vi "RF Test.vi"(0 "instrument handle":refnum<k15>, 2 "No Reverse":bool, 3 "file name":string, 5 "Num of Frames":i32, 9 "Num of Vectors":i32, 11 "error out":errorcluster) -> ()   [LabVIEW 2022 SP3]
uses:
  Motion Controllers/-MotionRoutines/MotionGlobals.vi
  <vilib>/Platform/TimedLoop/XDataNode/XDataNode.xnode
  <vilib>/Platform/TimedLoop/XDataNode/nitl_modes.ctl
  <vilib>/Platform/TimedLoop/XDataNode/XDNodeRunTimeDep.lvlib
  <vilib>/Platform/TimedLoop/XDataNode/wakeup.ctl
  <vilib>/Platform/TimedLoop/XDataNode/timing_clust.ctl
  <instrlib>/niScope/Acquire/Fetch/niScope Multi Fetch Binary 8.vi
  -ScanSystem/DataHandling/ReverseDataI8.vi
  Acqiris/-AcqirisRoutines/VScaleInfoAcq.vi
panel:
  in  "instrument handle 3":refnum<k15>
  out "x-y":u32
  out "result":i32
  in  "instrument handle 2":refnum<k15>
  out "frame time":u32
  out "Records Done":i32
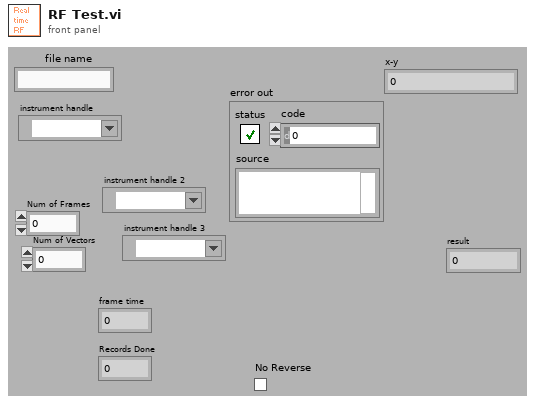
[diagram p1: front panel]
types:
  T1 = typedef "XDNodeRunTimeDep.lvlib/timing_clust.ctl" = cluster{"Expected End [f-1]":u64, "Actual End [f-1]":u64, "Finished Late? [f-1]":bool, "Expected End [i-1]":u64, "Actual End [i-1]":u64, "Finished Late? [i-1]":bool, "Expected Start [i]":u64, "Actual Start [i]":u64, "Expected Start [f]":u64, "Actual Start [f]":u64, "Source Name":string, "Structure Name":string, "Period":i64, "Deadline":i64, "Offset":i64, "Start":i64, "Priority":i32, "Timeout":i32, "Mode":T2, "Wakeup Reason":T3, "Error":errorcluster, "Source Type":string, "Secondary Source Type":string, "Global End Time":u64, "Global Start Time":u64, "Frame Duration":u64, "Iteration Duration":u64, "Assigned CPU":i32, "I/O Scan Engine Mode":u32}
  T2 = typedef "XDNodeRunTimeDep.lvlib/nitl_modes.ctl" = enum32{"No Change", "Process missed periods, maintain original phase", "Discard missed periods, maintain original phase", "Process missed periods, ignore original phase", "Discard missed periods, ignore original phase"}
  T3 = typedef "XDNodeRunTimeDep.lvlib/wakeup.ctl" = enum32{"Normal", "Aborted", "Asynchronous wakeup", "Timing source error", "Timed loop error", "Timeout"}
  T4 = cluster{sgl, "Gain [dB]  ":sgl, "Atten (dB)":sgl}
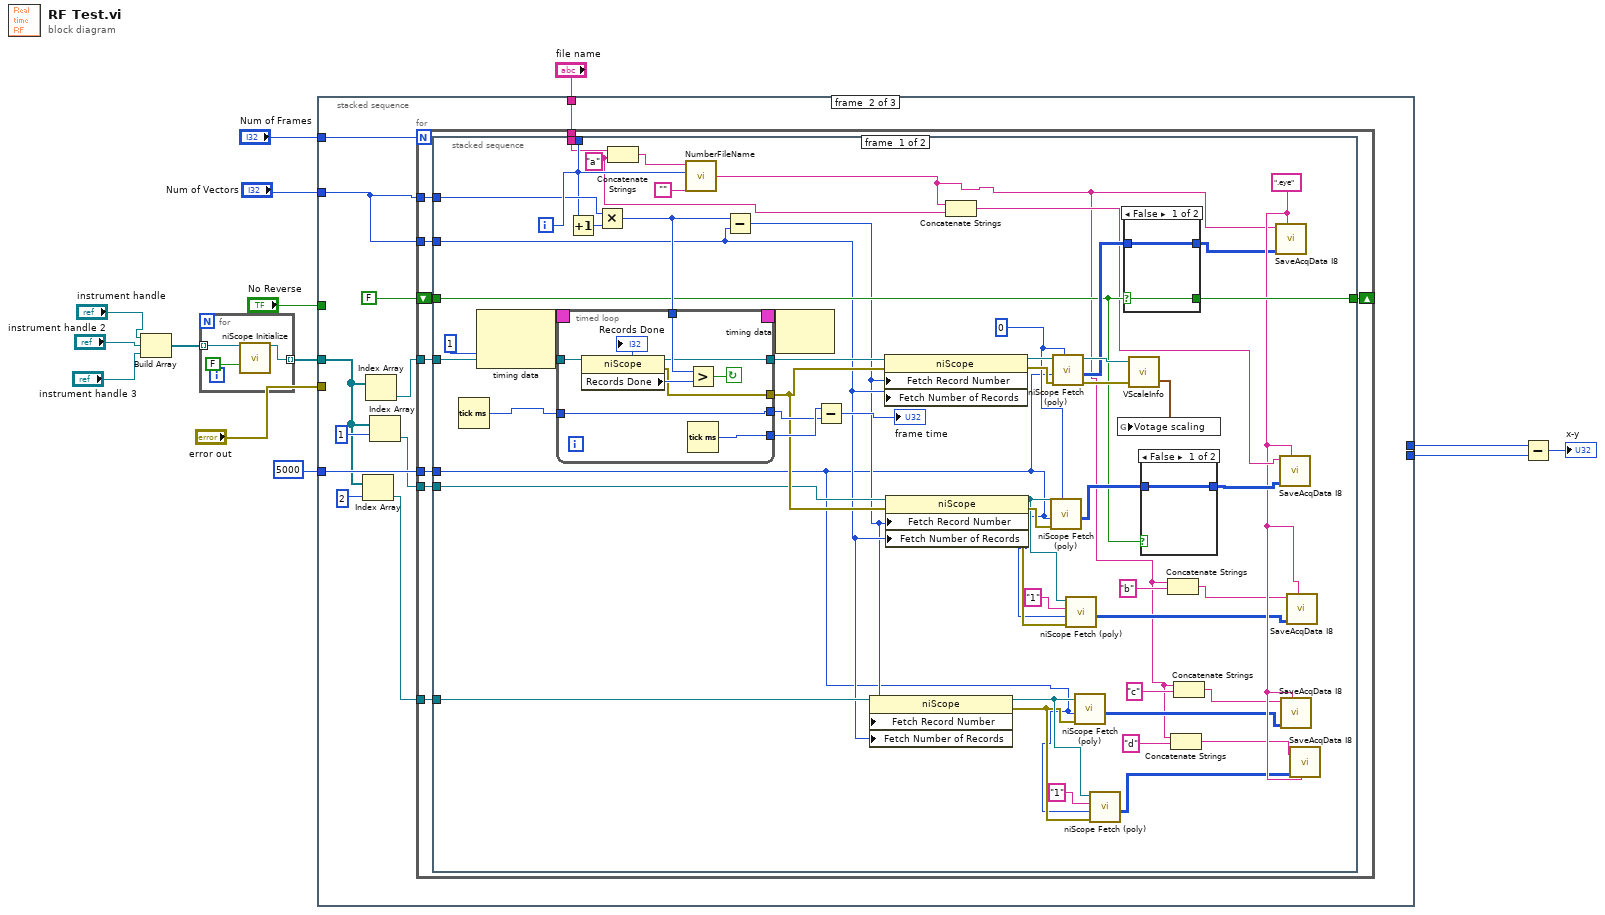
[diagram p0: block diagram]
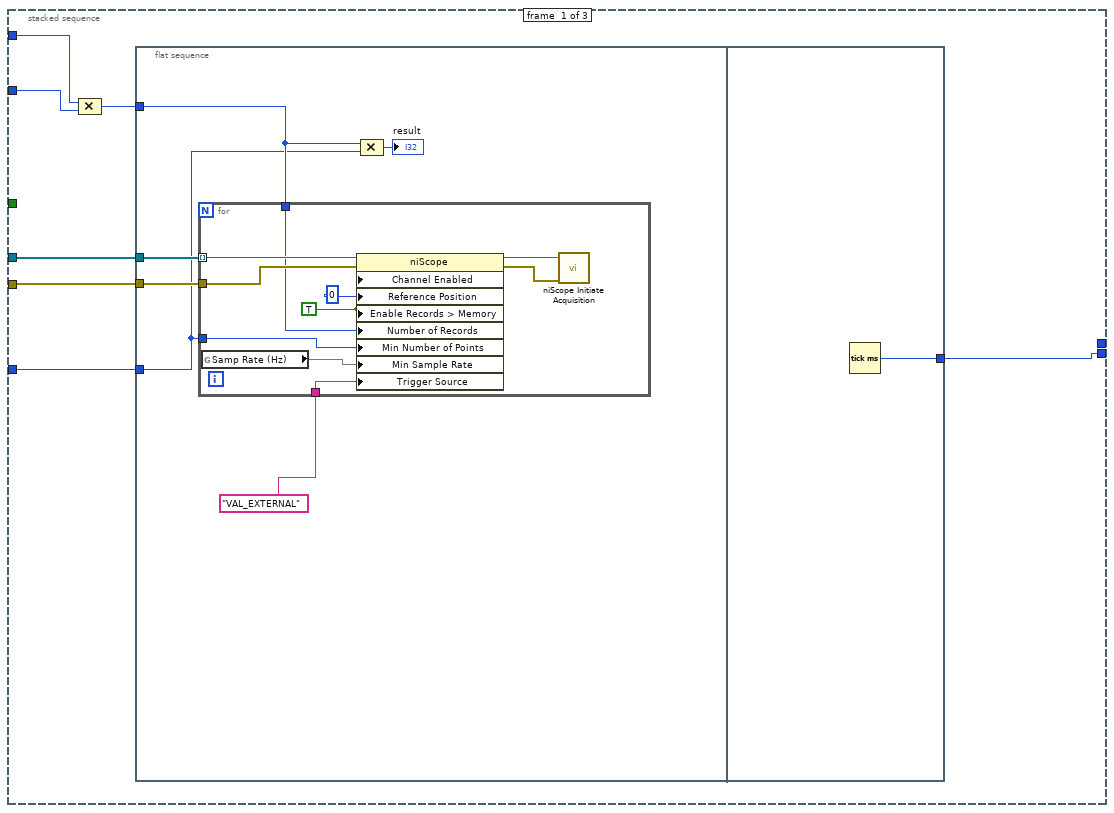
[diagram p2: hidden frame]
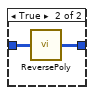
[diagram p3: hidden frame]
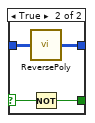
[diagram p4: hidden frame]
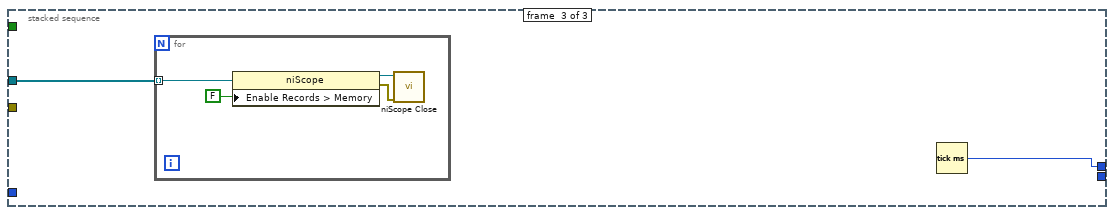
[diagram p6: hidden frame]
diagram:
  n1 = Build Array("instrument handle", "instrument handle 2", "instrument handle 3") -> (w2:refnum<k15>[])
  n2 = for {
    tunnel: [w17] -> w8 mode=indexing
    tunnel: w2 -> [w15] mode=indexing
    n3 = call <instrlib>:"niScope Initialize.vi"("resource name"=w15, "reset device"=FALSE) -> ("instrument handle"=w17:refnum<k15>)  [unwired: 2 in, 11 out]
  }
  n4 = stacked-sequence {
    tunnel: "error out" -> [w24 _ _]
    tunnel: w8 -> [w23 w44 w140]
    tunnel: "Num of Frames" -> [w22 w51 _]
    tunnel: "Num of Vectors" -> [w21 w48 _]
    tunnel: 5000 ("rf points per line") -> [w19 w52 _]
    tunnel: "file name" -> [_ w50 _]
    tunnel: "No Reverse" -> [_ _ _]
    tunnel: [_ _ w139] -> w7
    tunnel: [w18 _ _] -> w6
    frame #0 {
      n5 = Compound Arithmetic op=MULTIPLY(w22, w21) -> (w20:i32)
      n6 = flat-sequence {
        tunnel: w24 -> [w30]
        tunnel: w23 -> [w29]
        tunnel: w20 -> [w27]
        tunnel: w19 -> [w26]
        tunnel: [w41] -> w18
        frame #0 {
          n7 = for {
            tunnel: w30 -> [w39]
            tunnel: w29 -> [w38] mode=indexing
            tunnel: "VAL_EXTERNAL" ("Triggering:Trigger Source") -> [w33]
            tunnel: w27 -> [w32]
            tunnel: w26 -> [w31]
            w36 = TRUE ("Horizontal:Enable Records > Memory")
            n8 = global read "MotionGlobals.vi" "Samp Rate (Hz)"() -> (w34)
            n9 = property class="niScope"(reference=w38, error in=w39, "Channel Enabled"=w36, "Reference Position"=0, "Enable Records > Memory"=w36, "Number of Records"=w32, "Min Number of Points"=w31, "Min Sample Rate"=w34, "Trigger Source"=w33) -> (reference out=w40:refnum<k15>, error out=w37:errorcluster)
            n10 = call <instrlib>:"niScope Initiate Acquisition.vi"("instrument handle"=w40, "error in"=w37) -> ()  [unwired: 14 out]
          }
          n11 = Compound Arithmetic op=MULTIPLY(w27, w26) -> (→"result":i32)
        }
        frame #1 {
          n12 = Tick Count (ms)() -> (millisecond timer value=w41:u32)
        }
      }
    }
    frame #1 {
      n13 = Index Array(array=w44, index=2) -> (element=w42:refnum<k15>)
      n14 = Index Array(array=w44) -> (element=w47:refnum<k15>)  [unwired: 1 in]
      n15 = Index Array(array=w44, index=1) -> (element=w43:refnum<k15>)
      n16 = for {
        N: w51 -> [_]
        tunnel: w52 -> [w55]
        tunnel: w47 -> [w62]
        tunnel: w48 -> [w61]
        tunnel: w48 -> [w57]
        tunnel: w50 -> [w59]
        shift-right: [w58] -> _
        shift-left: FALSE -> [w56]
        tunnel: w43 -> [w54]
        tunnel: w42 -> [w53]
        i -> [w60]
        n17 = stacked-sequence {
          tunnel: w62 -> [w111 _]
          tunnel: w61 -> [w109 _]
          tunnel: w60 -> [w103 _]
          tunnel: w59 -> [w101 _]
          tunnel: [w98 _] -> w58
          tunnel: w57 -> [w80 _]
          tunnel: w56 -> [w92 _]
          tunnel: w55 -> [w78 _]
          tunnel: w54 -> [w84 _]
          tunnel: w53 -> [w81 _]
          frame #0 {
            w90 = 0
            w71 = ".eye" ("Ext")
            w91 = "a"
            n18 = Tick Count (ms)() -> (millisecond timer value=w88:u32)
            n19 = node-c288(i64 1 ("Period")) -> (w115:T1)  [unwired: 1 out]
            n20 = Increment(x=w103) -> (x+1=w110:i32)
            n21 = Multiply(x=w109, y=w110) -> (x*y=w106:i32)
            n22 = timed-loop {
              tunnel: w111 -> [w132]
              tunnel: w106 -> [w131]
              tunnel: [w129] -> w108
              tunnel: [w127] -> w89
              timing: w115 -> [_]
              timing-out: [_] -> w114
              tunnel: [w126] -> w95
              tunnel: w88 -> [w126]
              tunnel: [w125] -> w96
              stop <- w130 continue-if-true
              n23 = property class="niScope"(reference=w132) -> (reference out=w129:refnum<k15>, error out=w127:errorcluster, "Records Done"=w128:i32)  [unwired: 1 in]
              "Records Done" <- w128
              n24 = Greater?(x=w131, y=w128) -> (0:w130:bool)
              n25 = Tick Count (ms)() -> (millisecond timer value=w125:u32)
            }
            n26 = Concatenate Strings(w101, w91) -> (w100:string)
            n27 = call "NumberFileName.vi"("String"="", "File number"=w103, "file name"=w100) -> ("Numbered File"=w66:string)  [unwired: 1 in]
            n28 = Subtract(x=w106, y=w80) -> (x-y=w79:i32)
            n29 = node-c288(w114) -> ()  [unwired: 1 out]
            n30 = Subtract(x=w96, y=w95) -> (x-y=→"frame time":u32)
            n31 = property class="niScope"(reference=w81, "Fetch Record Number"=w79, "Fetch Number of Records"=w80) -> (reference out=w83:refnum<k15>, error out=w82:errorcluster)  [unwired: 1 in]
            n32 = property class="niScope"(reference=w108, error in=w89, "Fetch Record Number"=w79, "Fetch Number of Records"=w80) -> (reference out=w107:refnum<k15>, error out=w105:errorcluster)
            n33 = property class="niScope"(reference=w84, error in=w89, "Fetch Record Number"=w79, "Fetch Number of Records"=w80) -> (reference out=w85:refnum<k15>, error out=w86:errorcluster)
            n34 = Concatenate Strings(w66, w91) -> (w73:string)
            n35 = call-poly <instrlib>:"niScope Fetch (poly).vi"("timeout"=w90, "error in"=w86, "numSamples"=w78, "instrument handle"=w85) -> ("wfm"=w93:i8[][])  [unwired: 1 in, 6 out]
            n36 = call-poly <instrlib>:"niScope Fetch (poly).vi"("timeout"=w90, "error in"=w105, "numSamples"=w78, "instrument handle"=w107) -> ("error out"=w102:errorcluster, "wfm"=w99:i8[][], "instrument handle out"=w113:refnum<k15>)  [unwired: 1 in, 4 out]
            n37 = call-poly <instrlib>:"niScope Fetch (poly).vi"("error in"=w86, "numSamples"=w78, "channels"="1", "instrument handle"=w85) -> ("wfm"=w68:i8[][])  [unwired: 1 in, 6 out]
            n38 = call-poly <instrlib>:"niScope Fetch (poly).vi"("error in"=w82, "numSamples"=w78, "instrument handle"=w83) -> ("wfm"=w69:i8[][])  [unwired: 2 in, 6 out]
            n39 = call-poly <instrlib>:"niScope Fetch (poly).vi"("error in"=w82, "numSamples"=w78, "channels"="1", "instrument handle"=w83) -> ("wfm"=w70:i8[][])  [unwired: 1 in, 6 out]
            n40 = case shown="False" w92 {
              selector: w92 -> [w119 w124]
              tunnel: [w120 w121] -> w67
              tunnel: w99 -> [w120 w122]
              tunnel: [w119 w123] -> w98
              frame False {
              }
              frame True {
                n41 = call-poly "ReversePoly.vi"("Array in"=w122) -> ("Array out"=w121:i8[][])
                n42 = Not(x=w124) -> (.not. x?=w123:bool)
              }
            }
            n43 = call-poly "VScaleInfo.vi"("Instrument ID"=w113, "error in (no error)"=w102) -> ("Voltage Scale"=w112:T4)  [unwired: 1 in, 7 out]
            n44 = global write "MotionGlobals.vi" "Votage scaling"(w112) -> ()
            n45 = case shown="False" w92 {
              tunnel: [w116 w117] -> w72
              tunnel: w93 -> [w116 w118]
              frame False {
              }
              frame True {
                n46 = call-poly "ReversePoly.vi"("Array in"=w118) -> ("Array out"=w117:i8[][])
              }
            }
            n47 = Concatenate Strings(w66, "b") -> (w65:string)
            n48 = Concatenate Strings(w66, "d") -> (w63:string)
            n49 = Concatenate Strings(w66, "c") -> (w64:string)
            n50 = call "SaveAcqData I8.vi"("File Name"=w66, "Array"=w67, "Ext"=w71) -> ()  [unwired: 2 in, 1 out]
            n51 = call "SaveAcqData I8.vi"("File Name"=w73, "Array"=w72, "Ext"=w71) -> ()  [unwired: 2 in, 1 out]
            n52 = call "SaveAcqData I8.vi"("File Name"=w64, "Array"=w69, "Ext"=w71) -> ()  [unwired: 2 in, 1 out]
            n53 = call "SaveAcqData I8.vi"("File Name"=w65, "Array"=w68, "Ext"=w71) -> ()  [unwired: 2 in, 1 out]
            n54 = call "SaveAcqData I8.vi"("File Name"=w63, "Array"=w70, "Ext"=w71) -> ()  [unwired: 2 in, 1 out]
          }
          frame #1 {
          }
        }
      }
    }
    frame #2 {
      n55 = for {
        tunnel: w140 -> [w144] mode=indexing
        n56 = property class="niScope"(reference=w144, "Enable Records > Memory"=FALSE ("Horizontal:Enable Records > Memory")) -> (reference out=w142:refnum<k15>, error out=w141:errorcluster)  [unwired: 1 in]
        n57 = call <instrlib>:"niScope Close.vi"("instrument handle"=w142, "error in"=w141) -> ()  [unwired: 14 out]
      }
      n58 = Tick Count (ms)() -> (millisecond timer value=w139:u32)
    }
  }
  n59 = Subtract(x=w7, y=w6) -> (x-y=→"x-y":u32)
